vi "equilibrium_measurements_autofocus_build_brute_force.vi"() -> ()   [LabVIEW 2019]
uses:
  <vilib>/userDefined/High Color/IMAQdx.ctl
  <vilib>/vision/driver/IMAQdx.llb/IMAQdx Attribute Type.ctl
  <vilib>/vision/Management.llb/Cast Image 2 Method.ctl
  <vilib>/DAQmx/write.llb/DAQmx Write (Digital Bool 1Line 1Point).vi
  <vilib>/DAQmx/write.llb/DAQmx Write (Analog DBL 1Chan 1Samp).vi
  <vilib>/DAQmx/read.llb/DAQmx Read (Analog DBL 1Chan 1Samp).vi
  <vilib>/Analysis/baseanly.llb/Mean (DBL).vi
  <vilib>/DAQmx/create/channels.llb/DAQmx Create Channel (AO-Voltage-Basic).vi
  <vilib>/DAQmx/miscellaneous.llb/DAQmx Fill In Error Info.vi
  <vilib>/DAQmx/create/channels.llb/DAQmx Create Channel (AI-Temperature-Thermocouple).vi
  <vilib>/DAQmx/create/channels.llb/DAQmx Create Channel (CO-Pulse Generation-Frequency).vi
  <vilib>/DAQmx/configure/timing.llb/DAQmx Timing (Implicit).vi
  <vilib>/DAQmx/create/channels.llb/DAQmx Create Channel (DO-Digital Output).vi
  <vilib>/vision/driver/NI_Vision_Acquisition_Software.lvlib
  <resource>/objmgr/imaqdx.rc
  <vilib>/vision/NI_Vision_Development_Module.lvlib
  <vilib>/Analysis/NI_AALBase.lvlib
  <resource>/objmgr/daqmx.rc
panel:
  in  "Execute autofocus":bool=TRUE
  in  "Step Signal \nOutput Line 3":tag="/Dev3/PFI2"
  in  "Step Pulse Train \nFrequency (Hz) 3":dbl=200.0 format="%.6f"
  in  "Step Signal \nOutput Line 2":tag="/Dev3/PFI2"
  in  "Step Pulse Train \nFrequency (Hz) 2":dbl=200.0 format="%.6f"
  out "Direction":bool
  in  "Direction Line":tag="Dev3/port1/line4"
  in  "Enable Drive":bool
  in  "Enable Line":tag="Dev3/port1/line1"
  in  "Step Signal \nOutput Line":tag="/Dev3/PFI2"
  in  "Step Pulse Train \nFrequency (Hz)":dbl=200.0 format="%.6f"
  out "Video":bool
  in  "Action":i32(listbox)
  out "meanIntensity":dbl[](array[numeric])
  out "varLaplacian":dbl[](array[numeric])
  out "mean":dbl
  out "variance":dbl
  out "Avg Intensity":dbl(graph)=4.716017316017316
  in  "Monitor focus":bool
  out "?":dbl(graph)=701.3672509340029
  in  "ROI":T1={"Global Rectangle"=[], "Contours"=[{"Contour Type"=0, "ROI Type"=3, "Points"=[231, 86, 235, 90]}, {"Contour Type"=0, "ROI Type"=3, "Points"=[193, 50, 270, 125]}]}
  in  "error in":errorcluster
  in  "File path for video":string="C:\\Users\\Aniket\\Desktop\\mCherry_calibration\\new_lens\\laser_calibration\\laser_and_heating\\"
  in  "Laser profile file path":path=path "C:/Users/Aniket/Desktop/mCherry_calibration/new_lens/laser_calibration/laser_profiles/new_profile.txt"
  in  "Trigger Laser":bool
  in  "Power Generator":refnum<visa-resource-name>="COM3"
  in  "Desired \nTemperature":dbl=20.0 format="%#_13g"
  in  "PID Control":bool
  in  "Image file path \n(Do not add specify file extension - set to png)":path=path "C:/Users/Aniket/Desktop/mCherry_calibration/new_lens/laser_calibration/laser_profiles.txt"
  out "Current \nTemperature":dbl format="%0.2f"
  out "?":dbl[](graph)=[37.63236695538445]
  out "error out 7":errorcluster
  out "error out 6":errorcluster
  out "error out 5":errorcluster
  out "Exposure Time":dbl
  in  "ON/OFF":bool
  out "error out 3":errorcluster
  in  "LED":dbl(slide) scale=0.0..10.0
  in  "Refresh":bool
  out "Record":bool
  out "Processed Frames per Second":dbl
  out "Acquired Frame Rate":dbl
  out "error out":errorcluster
  out "Camera Display":T2(plugin-control) caption="Image Out"
  in  "Frame Rate":dbl=20.0
  out "Attribute Information Array":T4(array[cluster])
  in  "Session In":T5="cam0"
  # "Spot motion"
  # "Stage motion"
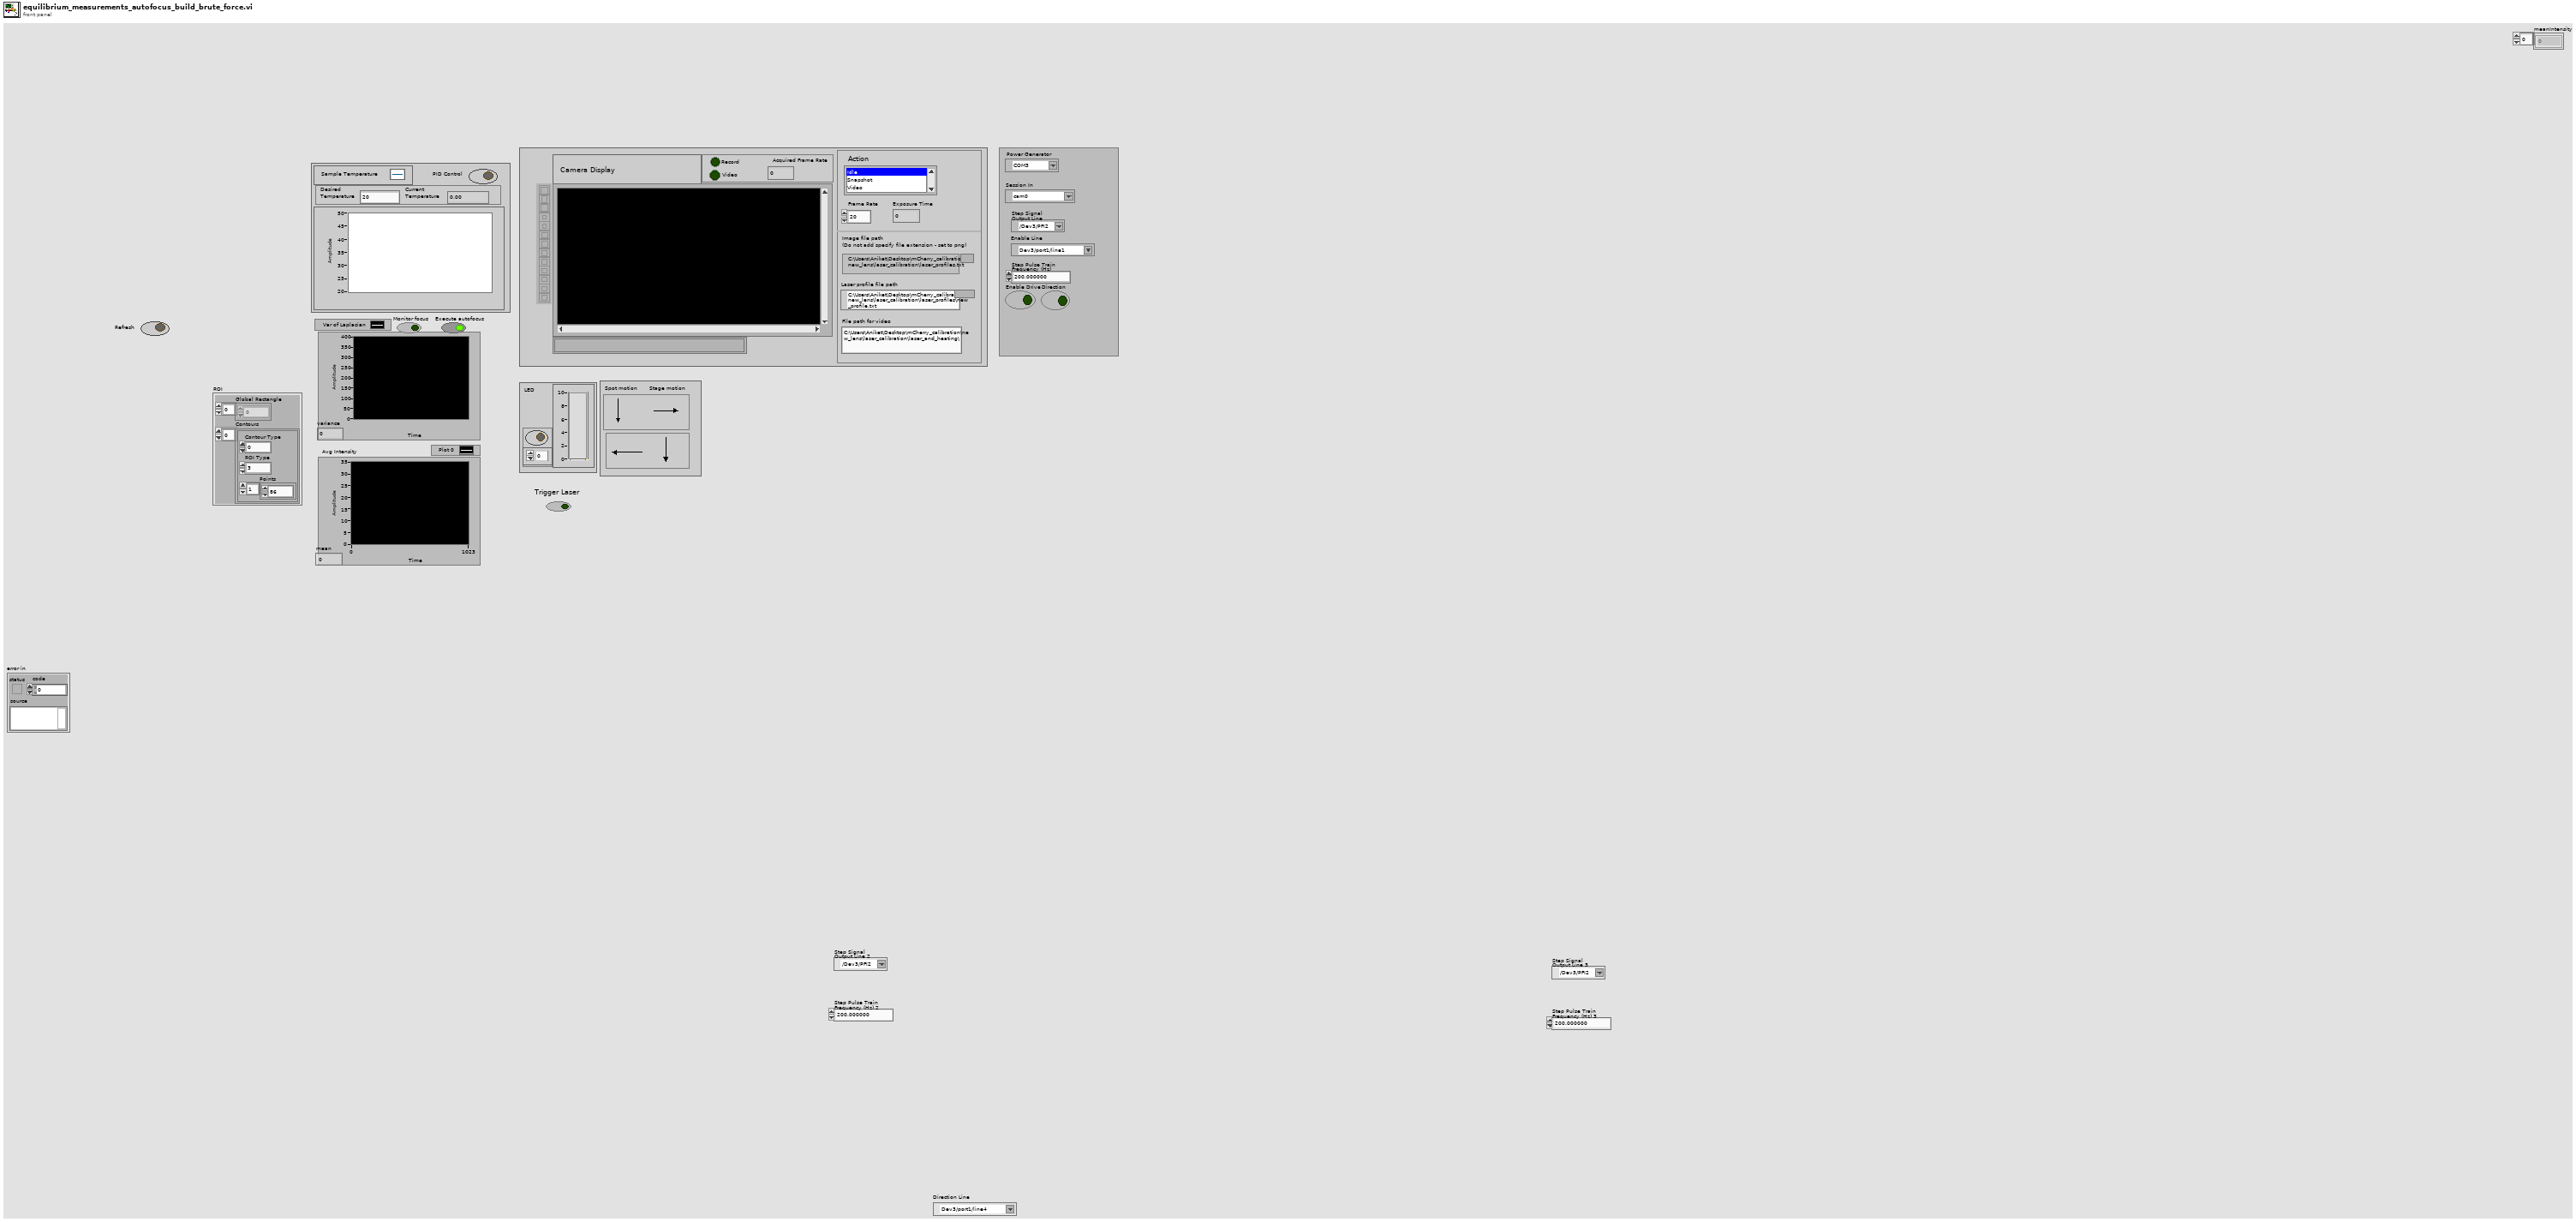
[diagram p1: front panel]
types:
  T1 = cluster{"Global Rectangle":i32[], "Contours":cluster{"Contour Type":u32, "ROI Type":u32, "Points":i32[]}[]}
  T2 = typedef "IMAQ Image.ctl" = refnum<image>
  T3 = typedef "NI_Vision_Acquisition_Software.lvlib/IMAQdx Attribute Type.ctl" = enum32{"U32", "I64", "DBL", "String", "Enum", "Bool", "Command"}
  T4 = cluster{"Attribute Type":T3, "Readable":bool, "Writable":bool, "Attribute Name":string}[]
  T5 = typedef "IMAQdx.ctl" = refnum<k21>
  T6 = typedef "Image Type" = u32
  T7 = typedef "ROI Descriptor" = cluster{"Global Rectangle":i32[], "Contours":cluster{"ID":enum32{"External", "Internal"}, "Type":u32, "Coordinates":i32[]}[]}
  T8 = typedef "IMAQ Rectangle" = cluster{"Left":i32, "Top":i32, "Right":i32, "Bottom":i32, "Rotation":dbl}
  T9 = cluster{"Mean Intensity":sgl, "Standard  Deviation":sgl, "Minimum Intensity":sgl, "Maximum Intensity":sgl}
  T10 = typedef "Cast Image 2 Method.ctl" = u32
  T11 = typedef "IMAQ AVI2 Refnum.ctl" = refnum<k20>
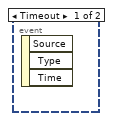
[diagram p3: hidden frame]
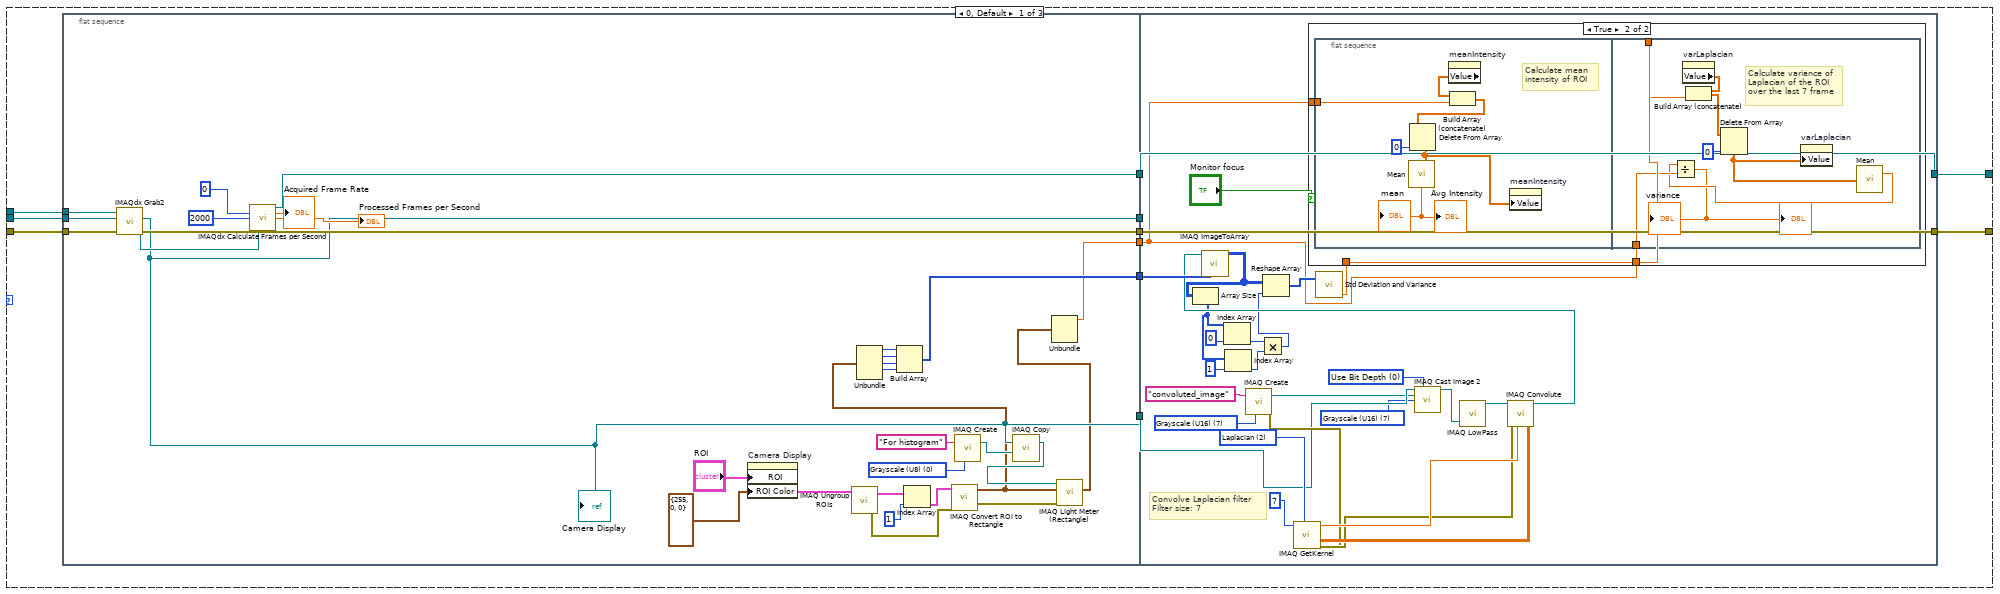
[diagram p6: hidden frame]
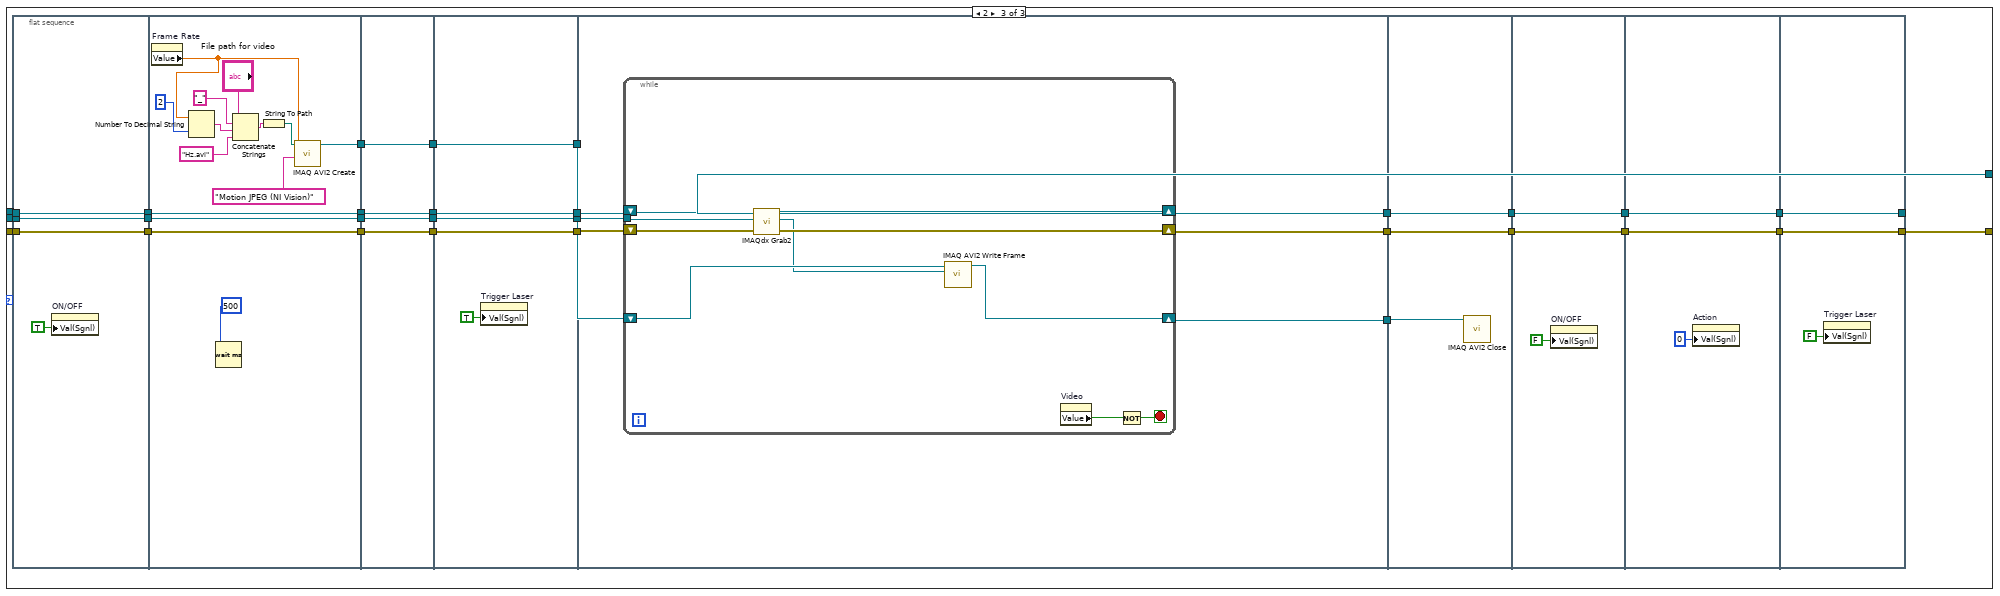
[diagram p8: hidden frame]
diagram:
  w12 = 10200 items=["Built-In"=10200, "Constant Value"=10116, "Channel"=10113]  # cjc source
  w14 = ""  # cjc channel
  w15 = 25.0  # cjc value
  w16 = 10072 items=["J"=10072, "K"=10073, "N"=10077, "R"=10082, "S"=10085, "T"=10086, "B"=10047, "E"=10055]  # thermocouple type
  w17 = 10143 items=["deg C"=10143, "deg F"=10144, "Kelvins"=10325, "deg R"=10145, "From Custom Scale"=10065]  # units
  w13 = "Temperature"  # channel name
  w18 = 0.0  # minimum value
  w19 = 100.0  # maximum value
  w21 = TRUE  # auto cleanup
  w44 = 10348 items=["Volts"=10348, "From Custom Scale"=10065] ("units")
  w46 = -1 items=["Default"=-1, "RSE"=10083, "NRSE"=10078, "Differential"=10106, "Pseudodifferential"=12529] ("input terminal configuration")
  w58 = T6 0 items=["Grayscale (U8)", "Grayscale (I16)", "Grayscale (SGL)", "Complex (CSG)", "RGB (U32)", "HSL (U32)", "RGB (U64)", "Grayscale (U16)"] ("Image Type")
  # "Total displacement of the objective from the origin\nMonitoring displacement allows keeping the search\nwithin a fixed range from the origin, to make sure\nthe objective does not drift too far"
  # "Set maximum exposure time \npermissible by the current frame rate"
  # "Excitation LED Control"
  # "Temperature measurement using thermocouple"
  # "PID Controller"
  # "Initialize arrays for focus detection"
  # "This array stores mean intensity in the last 10 frames\nInitiated as zeros"
  # "This array stores variance of Laplacian in the last 10 frames\nInitiated as zeros"
  n1 = call <vilib>:"DAQmx Create Task.vi"("auto cleanup"=w21, "error in"="error in") -> ("task out"=w20:refnum<k21>, "error out"=w22:errorcluster)  [unwired: 12 in]
  n2 = call-poly <vilib>:"DAQmx Create Virtual Channel.vi"("task in"=w20, "maximum value"=w19, "minimum value"=w18, "physical channels"=tag "Dev1/ai0", "cjc source"=w12, "name to assign"=w13, "units"=w17, "cjc channel"=w14, "error in"=w22, "thermocouple type"=w16, "cjc value"=w15) -> ("task out"=w11:refnum<k21>, "error out"=w10:errorcluster)  [unwired: 3 in]
  "error out 7" <- w10
  n3 = call-poly <vilib>:"DAQmx Create Virtual Channel.vi"("maximum value"=10.0, "minimum value"=0.0, "output terminal configuration"=w46, "physical channels"=tag "Dev3/ao0", "name to assign"="LED", "units"=w44) -> ("task out"=w42:refnum<k21>, "error out"=w41:errorcluster)  [unwired: 8 in]
  n4 = call <vilib>:"DAQmx Start Task.vi"("task/channels in"=w42, "error in"=w41) -> ("task out"=w40:refnum<k21>, "error out"=w39:errorcluster)  [unwired: 12 in]
  n5 = while {
    tunnel: w11 -> [w71]
    tunnel: w10 -> [w70]
    tunnel: [w69] -> w26
    tunnel: [w68] -> w25
    stop <- FALSE ("Monitor Temperature") stop-if-true
    n6 = Wait Until Next ms Multiple(millisecond multiple=u32 1000 ("millisecond timer value")) -> ()  [unwired: 1 out]
    n7 = call-poly <vilib>:"DAQmx Read.vi"("task/channels in"=w71, "error in"=w70) -> ("task out"=w69:refnum<k21>, "data"=w65:dbl, "error out"=w68:errorcluster)  [unwired: 11 in]
    n8 = Build Array(w65) -> (→"?":dbl[])
    n9 = Multiply(x=w65, y=1.07) -> (x*y=w63:dbl)
    n10 = Subtract(x=w63, y=2.74) -> (x-y=→"Current \nTemperature":dbl)
  }
  n11 = while {
    shift-right: [w75] -> w38
    shift-left: w40 -> [w77]
    shift-right: [w74] -> w37
    shift-left: w39 -> [w76]
    stop <- FALSE stop-if-true
    n12 = event shown="[0] \"LED\", \"ON/OFF\": Value Change" {
      selector: _ -> [_]
      dyn-events: _ -> [_]
      timeout: _ -> [_]
      tunnel: w77 -> [w86]
      tunnel: w76 -> [w85]
      tunnel: [w84] -> w75
      tunnel: [w83] -> w74
      event "LED", "ON/OFF": Value Change {
        n13 = event-data() -> ()  [unwired: 1 in, 6 out]
        n14 = Boolean To (0,1)(Boolean="ON/OFF") -> (0, 1=w79:i16)
        n15 = Multiply(x="LED", y=w79) -> (x*y=w78:dbl)
        n16 = call-poly <vilib>:"DAQmx Write.vi"("task/channels in"=w86, "auto start"=TRUE, "data"=w78, "error in"=w85) -> ("task out"=w84:refnum<k21>, "error out"=w83:errorcluster)  [unwired: 9 in, 1 out]
      }
    }
  }
  n17 = call "IMAQ Create"("Image Name"="Live", "Image Type"=w58) -> ("New Image"=w52:T2, "error out"=w51:errorcluster)  [unwired: 3 in]
  n18 = call <vilib>:"DAQmx Stop Task.vi"("task/channels in"=w26, "error in"=w25) -> ("error out"=→"error out 6":errorcluster)  [unwired: 12 in, 1 out]
  n19 = call <vilib>:"DAQmx Stop Task.vi"("task/channels in"=w38, "error in"=w37) -> ("error out"=→"error out 3":errorcluster)  [unwired: 12 in, 1 out]
  n20 = call <vilib>:"IMAQdx Open Camera.vi"("error in"=w51, "Session In"="Session In") -> ("error out"=w56:errorcluster, "Session Out"=w57:T5)  [unwired: 8 in]
  "error out 5" <- w56
  n21 = call <vilib>:"IMAQdx Enumerate Attributes.vi"("error in"=w56, "Session In"=w57) -> ("Attribute Information Array"=→"Attribute Information Array":T4)  [unwired: 7 in, 2 out]
  n22 = while {
    stop <- FALSE stop-if-true
    n23 = event shown="[1] \"Trigger Laser\": Value Change" {
      selector: _ -> [_ _]
      dyn-events: _ -> [_ _]
      timeout: _ -> [_ _]
      event Timeout {
        n24 = event-data() -> ()  [unwired: 1 in, 3 out]
      }
      event "Trigger Laser": Value Change {
        n25 = event-data() -> ()  [unwired: 1 in, 6 out]
        n26 = property on="Action" class="LstBox (strict)"() -> ("Value"=w88:i32)  [unwired: 2 in, 2 out]
        n27 = case shown="2" w88 {
          frame 0, Default {
          }
          frame 1 {
          }
          frame 2 {
            n28 = flat-sequence {
              frame #0 {
                "Video" <- TRUE ("Video")
              }
              frame #1 {
                # "Read voltage values for\nlaser control from a text file"
                n29 = Read from Text File(file (use dialog)="Laser profile file path") -> (text=w97:string)  [unwired: 3 in, 3 out]
                n30 = Spreadsheet String To Array(delimiter (Tab)="\r\n", format string="%f", spreadsheet string=w97, array type (2D Dbl)=dbl[][] []) -> (array=w99:dbl[][])
                n31 = Array Size(array=w99) -> (size(s)=w98:i32[])
                n32 = Index Array(array=w98, index=0) -> (element=w101:i32)
                n33 = Reshape Array(w99, w101) -> (w100:dbl[])
                n34 = call "Untitled 43.vi"() -> ("error out"=w90:errorcluster, "task out"=w91:refnum<k21>)  [unwired: 10 in]
                n35 = for {
                  N: w101 -> [_]
                  tunnel: w100 -> [w102] mode=indexing
                  tunnel: w91 -> [w104]
                  tunnel: w90 -> [w103]
                  w105 = TRUE  # auto start
                  n36 = Wait (ms)(milliseconds to wait=u32 10) -> ()  [unwired: 1 out]
                  n37 = call-poly <vilib>:"DAQmx Write.vi"("task/channels in"=w104, "auto start"=w105, "data"=w102, "error in"=w103) -> ()  [unwired: 9 in, 3 out]
                }
              }
              frame #2 {
                n38 = property on="Video" class="Bool (strict)"("Val(Sgnl)"=FALSE ("Value (Signaling)")) -> ()  [unwired: 2 in, 2 out]
              }
            }
          }
        }
      }
    }
  }
  n39 = while {
    stop <- FALSE stop-if-true
    n40 = local read "Current \nTemperature"() -> (w111:dbl)
    n41 = call "IronFishPIDtakeCurrentTemp.vi"(0:"Power Generator", "Switch"="PID Control", "Desired Temp"="Desired \nTemperature", "Current Temp"=w111) -> ()  [unwired: 4 in, 1 out]
  }
  n42 = while {
    stop <- FALSE stop-if-true
    n43 = event shown="[0] \"Execute autofocus\": Value Change" {
      selector: _ -> [_]
      dyn-events: _ -> [_]
      timeout: _ -> [_]
      event "Execute autofocus": Value Change {
        n44 = event-data() -> ()  [unwired: 1 in, 6 out]
        n45 = property on="Execute autofocus" class="Bool (strict)"() -> ("Value"=w114:bool)  [unwired: 2 in, 2 out]
        n46 = case shown="True" w114 {
          frame False {
          }
          frame True {
            # "Generate continuous samples for constant velocity, or finite \nsamples to move the motor a finite number of steps."
            # "Default is the\nobjective going\ndownwards"
            n47 = flat-sequence {
              tunnel: [w191] -> w117
              tunnel: w117 -> [w224]
              tunnel: [w224] -> w116
              tunnel: w116 -> [w226]
              frame #0 {
                n48 = flat-sequence {
                  tunnel: [w163] -> w158
                  tunnel: [w162] -> w157
                  tunnel: [w161] -> w154
                  tunnel: w158 -> [w183]
                  tunnel: w157 -> [w182]
                  tunnel: [w181] -> w156
                  tunnel: [w180] -> w155
                  tunnel: w154 -> [w179]
                  tunnel: w156 -> [w185]
                  tunnel: w155 -> [w184]
                  frame #0 {
                    n49 = property on="Direction" class="Bool (strict)"("Value"=FALSE ("Direction")) -> ()  [unwired: 2 in, 2 out]
                    n50 = Wait (ms)(milliseconds to wait=u32 50) -> ()  [unwired: 1 out]
                  }
                  frame #1 {
                    w164 = 150 ("samples per channel")
                    w176 = 10178 items=["Finite Samples"=10178, "Continuous Samples"=10123, "Hardware Timed Single Point"=12522] ("sample mode")
                    n51 = call-poly <vilib>:"DAQmx Create Virtual Channel.vi"("frequency"="Step Pulse Train \nFrequency (Hz) 2", "counter"=tag "Dev3/ctr0") -> ("task out"=w172:refnum<k21>, "error out"=w171:errorcluster)  [unwired: 12 in]
                    n52 = property class="DAQmx Channel"(reference=w172, error in=w171, "CO.Pulse.Term"="Step Signal \nOutput Line 2") -> (reference out=w175:refnum<k21>, error out=w174:errorcluster)
                    n53 = Divide(x=1000.0, y="Step Pulse Train \nFrequency (Hz) 2") -> (x/y=w167:dbl)
                    n54 = Multiply(x=w167, y=w164) -> (x*y=w169:dbl)
                    n55 = Add(x=w169, y=5.0) -> (x+y=w161:dbl)
                    n56 = call-poly <vilib>:"DAQmx Timing.vi"("task/channels in"=w175, "sample mode"=w176, "samples per channel"=w164, "error in"=w174) -> ("task out"=w178:refnum<k21>, "error out"=w177:errorcluster)  [unwired: 10 in]
                    n57 = call <vilib>:"DAQmx Start Task.vi"("task/channels in"=w178, "error in"=w177) -> ("task out"=w163:refnum<k21>, "error out"=w162:errorcluster)  [unwired: 12 in]
                  }
                  frame #2 {
                    n58 = call <vilib>:"DAQmx Is Task Done.vi"("task/channels in"=w183, "error in"=w182) -> ("task out"=w180:refnum<k21>, "error out"=w181:errorcluster)  [unwired: 11 in, 1 out]
                    n59 = Wait (ms)(milliseconds to wait=w179) -> ()  [unwired: 1 out]
                  }
                  frame #3 {
                    n60 = call <vilib>:"DAQmx Stop Task.vi"("task/channels in"=w184, "error in"=w185) -> ("task out"=w188:refnum<k21>, "error out"=w186:errorcluster)  [unwired: 12 in]
                    n61 = call <vilib>:"DAQmx Clear Task.vi"("task in"=w188, "error in"=w186) -> ("error out"=w187:errorcluster)  [unwired: 13 in]
                    n62 = call <vilib>:"Simple Error Handler.vi"("error in (no error)"=w187) -> ()  [unwired: 4 in, 5 out]
                  }
                }
              }
              frame #1 {
                n63 = property on="Direction" class="Bool (strict)"("Value"=TRUE ("Direction")) -> ()  [unwired: 2 in, 2 out]
                n64 = Wait (ms)(milliseconds to wait=u32 50) -> ()  [unwired: 1 out]
              }
              frame #2 {
                # "Note that coincidentally,\nthe gradient and the number\nof steps is numerically the same"
                n65 = for {
                  N: 450 -> [_]
                  tunnel: [w196] -> w194 mode=indexing
                  n66 = flat-sequence {
                    tunnel: [w221] -> w196
                    frame #0 {
                      w211 = 10178 items=["Finite Samples"=10178, "Continuous Samples"=10123, "Hardware Timed Single Point"=12522] ("sample mode")
                      n67 = call-poly <vilib>:"DAQmx Create Virtual Channel.vi"("frequency"="Step Pulse Train \nFrequency (Hz)", "counter"=tag "Dev3/ctr0") -> ("task out"=w203:refnum<k21>, "error out"=w202:errorcluster)  [unwired: 12 in]
                      n68 = Divide(x=1000.0, y="Step Pulse Train \nFrequency (Hz)") -> (x/y=w206:dbl)
                      n69 = property class="DAQmx Channel"(reference=w203, error in=w202, "CO.Pulse.Term"="Step Signal \nOutput Line") -> (reference out=w210:refnum<k21>, error out=w209:errorcluster)
                      n70 = Multiply(x=w206, y=1.0) -> (x*y=w208:dbl)
                      n71 = Add(x=w208, y=2.0) -> (x+y=w214:dbl)
                      n72 = Wait (ms)(milliseconds to wait=w214) -> ()  [unwired: 1 out]
                      n73 = call-poly <vilib>:"DAQmx Timing.vi"("task/channels in"=w210, "sample mode"=w211, "samples per channel"=1, "error in"=w209) -> ("task out"=w213:refnum<k21>, "error out"=w212:errorcluster)  [unwired: 10 in]
                      n74 = call <vilib>:"DAQmx Start Task.vi"("task/channels in"=w213, "error in"=w212) -> ("task out"=w216:refnum<k21>, "error out"=w215:errorcluster)  [unwired: 12 in]
                      n75 = call <vilib>:"DAQmx Is Task Done.vi"("task/channels in"=w216, "error in"=w215) -> ("task out"=w219:refnum<k21>, "error out"=w218:errorcluster)  [unwired: 11 in, 1 out]
                      n76 = call <vilib>:"DAQmx Stop Task.vi"("task/channels in"=w219, "error in"=w218) -> ("task out"=w220:refnum<k21>, "error out"=w217:errorcluster)  [unwired: 12 in]
                      n77 = call <vilib>:"DAQmx Clear Task.vi"("task in"=w220, "error in"=w217) -> ("error out"=w198:errorcluster)  [unwired: 13 in]
                      n78 = call <vilib>:"Simple Error Handler.vi"("error in (no error)"=w198) -> ()  [unwired: 4 in, 5 out]
                    }
                    frame #1 {
                      n79 = property on="variance" class="DigNum (strict)"() -> ("Value"=w221:dbl)  [unwired: 2 in, 2 out]
                    }
                  }
                }
                n80 = Array Max & Min(array=w194) -> (max index (indices)=w193:i32)  [unwired: 3 out]
                n81 = Subtract(x=449, y=w193) -> (x-y=w191:i32)
              }
              frame #3 {
                n82 = property on="Direction" class="Bool (strict)"("Value"=FALSE ("Direction")) -> ()  [unwired: 2 in, 2 out]
                n83 = Wait (ms)(milliseconds to wait=u32 50) -> ()  [unwired: 1 out]
              }
              frame #4 {
                # "offset"
                n84 = flat-sequence {
                  tunnel: w227 -> [w236]
                  tunnel: [w235] -> w232
                  tunnel: [w234] -> w231
                  tunnel: [w233] -> w228
                  tunnel: w232 -> [w255]
                  tunnel: w231 -> [w254]
                  tunnel: [w253] -> w230
                  tunnel: [w252] -> w229
                  tunnel: w228 -> [w251]
                  tunnel: w230 -> [w257]
                  tunnel: w229 -> [w256]
                  frame #0 {
                    w248 = 10178 items=["Finite Samples"=10178, "Continuous Samples"=10123, "Hardware Timed Single Point"=12522] ("sample mode")
                    n85 = call-poly <vilib>:"DAQmx Create Virtual Channel.vi"("frequency"="Step Pulse Train \nFrequency (Hz) 3", "counter"=tag "Dev3/ctr0") -> ("task out"=w240:refnum<k21>, "error out"=w239:errorcluster)  [unwired: 12 in]
                    n86 = Divide(x=1000.0, y="Step Pulse Train \nFrequency (Hz) 3") -> (x/y=w243:dbl)
                    n87 = property class="DAQmx Channel"(reference=w240, error in=w239, "CO.Pulse.Term"="Step Signal \nOutput Line 3") -> (reference out=w247:refnum<k21>, error out=w246:errorcluster)
                    n88 = Multiply(x=w243, y=w236) -> (x*y=w245:dbl)
                    n89 = Add(x=w245, y=5.0) -> (x+y=w233:dbl)
                    n90 = call-poly <vilib>:"DAQmx Timing.vi"("task/channels in"=w247, "sample mode"=w248, "samples per channel"=w236, "error in"=w246) -> ("task out"=w250:refnum<k21>, "error out"=w249:errorcluster)  [unwired: 10 in]
                    n91 = call <vilib>:"DAQmx Start Task.vi"("task/channels in"=w250, "error in"=w249) -> ("task out"=w235:refnum<k21>, "error out"=w234:errorcluster)  [unwired: 12 in]
                  }
                  frame #1 {
                    n92 = call <vilib>:"DAQmx Is Task Done.vi"("task/channels in"=w255, "error in"=w254) -> ("task out"=w253:refnum<k21>, "error out"=w252:errorcluster)  [unwired: 11 in, 1 out]
                    n93 = Wait (ms)(milliseconds to wait=w251) -> ()  [unwired: 1 out]
                  }
                  frame #2 {
                    n94 = call <vilib>:"DAQmx Stop Task.vi"("task/channels in"=w257, "error in"=w256) -> ("task out"=w260:refnum<k21>, "error out"=w259:errorcluster)  [unwired: 12 in]
                    n95 = call <vilib>:"DAQmx Clear Task.vi"("task in"=w260, "error in"=w259) -> ("error out"=w258:errorcluster)  [unwired: 13 in]
                    n96 = call <vilib>:"Simple Error Handler.vi"("error in (no error)"=w258) -> ()  [unwired: 4 in, 5 out]
                  }
                }
                n97 = Subtract(x=w226, y=20) -> (x-y=w227:i32)
              }
              frame #5 {
                n98 = property on="Execute autofocus" class="Bool (strict)"("Val(Sgnl)"=FALSE ("Value (Signaling)")) -> ()  [unwired: 2 in, 2 out]
              }
            }
            n99 = while {
              stop <- w118 stop-if-true
              (unwired) FALSE
              w121 = 0 items=["one channel for each line", "one channel for all lines"] ("line grouping")
              w120 = 0 items=["one channel for each line", "one channel for all lines"] ("line grouping")
              # "Direction Line"
              # "Enable lines"
              n100 = call-poly <vilib>:"DAQmx Create Virtual Channel.vi"("lines"="Enable Line", "line grouping"=w120) -> ("task out"=w134:refnum<k21>, "error out"=w135:errorcluster)  [unwired: 12 in]
              n101 = call-poly <vilib>:"DAQmx Create Virtual Channel.vi"("lines"="Direction Line", "line grouping"=w121) -> ("task out"=w130:refnum<k21>, "error out"=w131:errorcluster)  [unwired: 12 in]
              n102 = flat-sequence {
                tunnel: w130 -> [w144]
                tunnel: w131 -> [w143]
                tunnel: [w142] -> w139
                tunnel: [w141] -> w138
                tunnel: [w152] -> w133
                tunnel: [w153] -> w132
                tunnel: w139 -> [w153]
                tunnel: w138 -> [w152]
                tunnel: w134 -> [w149]
                tunnel: w135 -> [w148]
                tunnel: [w147] -> w136
                tunnel: [w146] -> w137
                frame #0 {
                  n103 = property on="Direction" class="Bool (strict)"() -> ("Value"=w140:bool)  [unwired: 2 in, 2 out]
                  n104 = call-poly <vilib>:"DAQmx Write.vi"("task/channels in"=w144, "auto start"=TRUE, "data"=w140, "error in"=w143) -> ("task out"=w142:refnum<k21>, "error out"=w141:errorcluster)  [unwired: 9 in, 1 out]
                }
                frame #1 {
                  n105 = call-poly <vilib>:"DAQmx Write.vi"("task/channels in"=w149, "auto start"=TRUE, "data"="Enable Drive", "error in"=w148) -> ("task out"=w147:refnum<k21>, "error out"=w146:errorcluster)  [unwired: 9 in, 1 out]
                }
              }
              n106 = call <vilib>:"DAQmx Stop Task.vi"("task/channels in"=w136, "error in"=w137) -> ("task out"=w123:refnum<k21>, "error out"=w124:errorcluster)  [unwired: 12 in]
              n107 = property on="Execute autofocus" class="Bool (strict)"() -> ("Value"=w119:bool)  [unwired: 2 in, 2 out]
              n108 = call <vilib>:"DAQmx Stop Task.vi"("task/channels in"=w132, "error in"=w133) -> ("task out"=w129:refnum<k21>, "error out"=w128:errorcluster)  [unwired: 12 in]
              n109 = call <vilib>:"DAQmx Clear Task.vi"("task in"=w123, "error in"=w124) -> ("error out"=w125:errorcluster)  [unwired: 13 in]
              n110 = Not(x=w119) -> (.not. x?=w118:bool)
              n111 = call <vilib>:"DAQmx Clear Task.vi"("task in"=w129, "error in"=w128) -> ("error out"=w127:errorcluster)  [unwired: 13 in]
              n112 = call <vilib>:"Simple Error Handler.vi"("error in (no error)"=w127) -> ()  [unwired: 4 in, 5 out]
              n113 = call <vilib>:"Simple Error Handler.vi"("error in (no error)"=w125) -> ()  [unwired: 4 in, 5 out]
            }
            "Direction" <- FALSE ("Clockwise/Counterclockwise?")
          }
        }
      }
    }
  }
  n114 = call <vilib>:"IMAQdx Configure Grab.vi"("error in"=w56, "Session In"=w57) -> ("error out"=w54:errorcluster, "Session Out"=w35:T5)  [unwired: 8 in]
  n115 = while {
    stop <- FALSE stop-if-true
    n116 = event shown="[0] \"Refresh\": Value Change" {
      selector: _ -> [_]
      dyn-events: _ -> [_]
      timeout: _ -> [_]
      event "Refresh": Value Change {
        (unwired) dbl[] [] ("History Data")
        n117 = event-data() -> ()  [unwired: 1 in, 4 out]
      }
    }
  }
  n118 = property class="IMAQdx"(reference=w35, error in=w54, "ActiveAttribute"="CameraAttributes::AcquisitionControl::AcquisitionFrameRate", "ValueDBL"="Frame Rate") -> (reference out=w30:T5, error out=w28:errorcluster)
  n119 = local write "Frame Rate"("Frame Rate") -> ()
  n120 = local read "Frame Rate"() -> (w32:dbl)
  n121 = Divide(x=991000.0, y=w32) -> (x/y=w31:dbl)
  "Exposure Time" <- w31
  n122 = property class="IMAQdx"(reference=w30, error in=w28, "ActiveAttribute"="CameraAttributes::AcquisitionControl::ExposureTime", "ValueDBL"=w31) -> (reference out=w29:T5, error out=w27:errorcluster)
  n123 = property on="Action" class="LstBox (strict)"("Val(Sgnl)"=0 ("Value (Signaling)")) -> ()  [unwired: 2 in, 2 out]
  n124 = while {
    tunnel: w29 -> [w269]
    tunnel: w52 -> [w267]
    shift-right: [w266] -> w50
    shift-left: w27 -> [w268]
    tunnel: [w263] -> w2
    stop <- FALSE ("Stop") stop-if-true
    n125 = case shown="1" "Action" {
      tunnel: w269 -> [w280 w372 w443]
      tunnel: w268 -> [w279 w374 w441]
      tunnel: w267 -> [w278 w373 w442]
      tunnel: [w277 w375 w439] -> w266
      tunnel: [w276 w376 w440] -> w263
      frame 0, Default {
        n126 = flat-sequence {
          tunnel: w280 -> [w310]
          tunnel: w279 -> [w309]
          tunnel: w278 -> [w308]
          tunnel: [w307] -> w275
          tunnel: [w305] -> w274
          tunnel: [w292] -> w273
          tunnel: [w292] -> w272
          tunnel: [w284] -> w271
          tunnel: [w281] -> w270
          tunnel: [w338] -> w276
          tunnel: [w339] -> w277
          tunnel: w275 -> [w339]
          tunnel: w274 -> [w338]
          tunnel: w273 -> [_]
          tunnel: w272 -> [w320]
          tunnel: w271 -> [w329]
          tunnel: w270 -> [w311]
          frame #0 {
            w293 = T6 0 items=["Grayscale (U8)", "Grayscale (I16)", "Grayscale (SGL)", "Complex (CSG)", "RGB (U32)", "HSL (U32)", "RGB (U64)", "Grayscale (U16)"] ("Image Type")
            n127 = call <vilib>:"IMAQdx Grab2.vi"("error in"=w309, "Image In"=w308, "Session In"=w310) -> ("error out"=w307:errorcluster, "Image Out"=w292:T2, "Session Out"=w306:T5)  [unwired: 5 in, 1 out]
            "Camera Display" <- w292
            n128 = call <vilib>:"IMAQdx Calculate Frames per Second.vi"("Session In"=w306, "Buffer Number"=u32 0, "Minimum Display Update Interval (ms)"=u32 2000) -> ("Session Out"=w305:T5, "Acquired Frames per Second"=→"Acquired Frame Rate":dbl, "Processed Frames per Second"=→"Processed Frames per Second":dbl)  [unwired: 6 in, 4 out]
            n129 = property on="Camera Display" class="ImageControl"("ROI"="ROI", "ROI Color"=cluster{"Red":u8, "Green":u8, "Blue":u8} {"Red"=255, "Green"=0, "Blue"=0}) -> ()  [unwired: 2 in, 2 out]
            n130 = call "IMAQ Ungroup ROIs"("ROI Descriptor"="ROI") -> ("error out"=w296:errorcluster, "ROI Descriptors out"=w299:T7[])  [unwired: 3 in]
            n131 = Index Array(array=w299, index=1) -> (element=w297:T7)
            n132 = call "IMAQ Convert ROI to Rectangle"("error in (no error)"=w296, "ROI Descriptor"=w297) -> ("error out"=w295:errorcluster, "Rectangle"=w289:T8)  [unwired: 7 in]
            n133 = Unbundle(w289) -> ("Left"=w288:i32, "Top"=w287:i32, "Right"=w286:i32, "Bottom"=w285:i32)  [unwired: 1 out]
            n134 = Build Array(w288, w287, w286, w285) -> (w284:i32[])
            n135 = call "IMAQ Create"("Image Name"="For histogram", "Image Type"=w293) -> ("New Image"=w291:T2)  [unwired: 3 in, 1 out]
            n136 = call "IMAQ Copy"("Image Dst"=w291, "Image Src"=w292) -> ("Image Dst Out"=w290:T2)  [unwired: 4 in, 1 out]
            n137 = call "IMAQ Light Meter (Rectangle)"("error in (no error)"=w295, "Rectangle"=w289, "Image"=w290) -> ("Gray Level Intensities"=w282:T9)  [unwired: 4 in, 4 out]
            n138 = Unbundle(w282) -> ("Mean Intensity"=w281:sgl)  [unwired: 3 out]
          }
          frame #1 {
            w316 = T6 7 items=["Grayscale (U8)", "Grayscale (I16)", "Grayscale (SGL)", "Complex (CSG)", "RGB (U32)", "HSL (U32)", "RGB (U64)", "Grayscale (U16)"] ("Image Type")
            w319 = T10 0 items=["Use Bit Depth", "Shift", "Use Lookup Table"] ("Method")
            w334 = u16 2 items=["Gradient"=1, "Laplacian"=2, "Smoothing"=3, "Gaussian"=4] ("Kernel Family")
            w336 = T6 7 items=["Grayscale (U8)", "Grayscale (I16)", "Grayscale (SGL)", "Complex (CSG)", "RGB (U32)", "HSL (U32)", "RGB (U64)", "Grayscale (U16)"] ("Image Type")
            # "Convolve Laplacian filter \nFilter size: 7"
            n139 = call "IMAQ Create"("Image Name"="convoluted_image", "Image Type"=w336) -> ("New Image"=w318:T2, "error out"=w330:errorcluster)  [unwired: 3 in]
            n140 = call "IMAQ GetKernel"("Kernel Family"=w334, "error in (no error)"=w330, "Kernel Size (3,5,...)"=7) -> ("error out"=w331:errorcluster, "Kernel"=w332:sgl[][], "Divider"=w333:sgl)  [unwired: 5 in, 1 out]
            n141 = call "IMAQ Cast Image 2"("Image Src"=w320, "Method"=w319, "Image Dst"=w318, "Image Type"=w316) -> ("Image Dst Out"=w317:T2)  [unwired: 10 in, 1 out]
            n142 = call "IMAQ LowPass"("Image Src"=w317) -> ("Image Dst Out"=w321:T2)  [unwired: 6 in, 1 out]
            n143 = call "IMAQ Convolute"("Kernel"=w332, "Divider (kernel sum)"=w333, "error in (no error)"=w331, "Image Src"=w321) -> ("Image Dst Out"=w328:T2)  [unwired: 6 in, 1 out]
            n144 = call "IMAQ ImageToArray"("Optional Rectangle"=w329, "Image"=w328) -> ("Image Pixels (U16)"=w312:u16[][])  [unwired: 2 in, 4 out]
            n145 = Array Size(array=w312) -> (size(s)=w315:i32[])
            n146 = Index Array(array=w315, index=0 ("index (row)")) -> (element=w325:i32)
            n147 = Index Array(array=w315, index=1) -> (element=w324:i32)
            n148 = Multiply(x=w325, y=w324) -> (x*y=w314:i32)
            n149 = Reshape Array(w312, w314) -> (w313:u16[])
            n150 = call <vilib>:"Std Deviation and Variance.vi"("X"=w313) -> ("variance"=w322:dbl)  [unwired: 1 in, 2 out]
            n151 = case shown="True" "Monitor focus" {
              tunnel: w322 -> [_ w342]
              tunnel: w311 -> [_ w341]
              tunnel: w311 -> [_ w340]
              frame False {
              }
              frame True {
                n152 = flat-sequence {
                  tunnel: w340 -> [w343]
                  tunnel: w342 -> [w352]
                  tunnel: w341 -> [w356]
                  frame #0 {
                    # "Calculate mean \nintensity of ROI"
                    n153 = property on="meanIntensity" class="Arr (strict)"() -> ("Value"=w346:dbl[])  [unwired: 2 in, 2 out]
                    n154 = Build Array (concatenate)(w346, w343) -> (w345:dbl[])
                    n155 = Delete From Array(array=w345, index=0) -> (array with subset deleted=w344:dbl[])  [unwired: 1 in, 1 out]
                    n156 = call-poly <vilib>:"Mean.vi"("X"=w344) -> ("mean"=→"Avg Intensity" →"mean":dbl)  [unwired: 1 out]
                    n157 = property on="meanIntensity" class="Arr (strict)"("Value"=w344) -> ()  [unwired: 2 in, 2 out]
                  }
                  frame #1 {
                    # "Calculate variance of\nLaplacian of the ROI\nover the last 7 frame"
                    n158 = property on="varLaplacian" class="Arr (strict)"() -> ("Value"=w353:dbl[])  [unwired: 2 in, 2 out]
                    n159 = Build Array (concatenate)(w353, w352) -> (w351:dbl[])
                    n160 = Delete From Array(array=w351, index=0) -> (array with subset deleted=w350:dbl[])  [unwired: 1 in, 1 out]
                    n161 = property on="varLaplacian" class="Arr (strict)"("Value"=w350) -> ()  [unwired: 2 in, 2 out]
                    n162 = call-poly <vilib>:"Mean.vi"("X"=w350) -> ("mean"=w355:dbl)  [unwired: 1 out]
                    n163 = Divide(x=w355, y=w356) -> (x/y=→"?" →"variance":dbl)
                  }
                }
              }
            }
          }
        }
      }
      frame 1 {
        n164 = flat-sequence {
          tunnel: w372 -> [w378]
          tunnel: w373 -> [w379]
          tunnel: w374 -> [w380]
          tunnel: [w380] -> w361
          tunnel: [w379] -> w360
          tunnel: [w378] -> w359
          tunnel: [w384] -> w367
          tunnel: [w383] -> w365
          tunnel: [w382] -> w363
          tunnel: w361 -> [w384]
          tunnel: w360 -> [w383]
          tunnel: w359 -> [w382]
          tunnel: w367 -> [w388]
          tunnel: [w388] -> w366
          tunnel: w365 -> [w387]
          tunnel: [w387] -> w364
          tunnel: w363 -> [w386]
          tunnel: [w386] -> w362
          tunnel: [w401] -> w371
          tunnel: [w405] -> w369
          tunnel: w366 -> [w404]
          tunnel: w364 -> [w403]
          tunnel: w362 -> [w402]
          tunnel: w371 -> [w408]
          tunnel: [w408] -> w370
          tunnel: w369 -> [w407]
          tunnel: [w407] -> w368
          tunnel: w370 -> [w411]
          tunnel: w368 -> [w410]
          tunnel: [w411] -> w358
          tunnel: [w410] -> w357
          tunnel: [w413] -> w375
          tunnel: [w414] -> w376
          tunnel: w358 -> [w414]
          tunnel: w357 -> [w413]
          frame #0 {
            "Record" <- TRUE ("Record")
          }
          frame #1 {
            n165 = property on="ON/OFF" class="Bool (strict)"("Val(Sgnl)"=TRUE ("ON/OFF")) -> ()  [unwired: 2 in, 2 out]
          }
          frame #2 {
            n166 = Wait (ms)(milliseconds to wait=u32 500) -> ()  [unwired: 1 out]
          }
          frame #3 {
            n167 = property on="Current \nTemperature" class="DigNum (strict)"() -> ("Value"=w399:dbl)  [unwired: 2 in, 2 out]
            n168 = Path To String(path="Image file path \n(Do not add specify file extension - set to png)") -> (string=w394:string)
            n169 = Number To Fractional String(number=w399, precision (6)=i16 2 ("width (-)")) -> (F-format string=w396:string)  [unwired: 2 in]
            n170 = Concatenate Strings("_" ("string"), w396) -> (w393:string)
            n171 = Concatenate Strings(w394, w393) -> (w392:string)
            n172 = call <vilib>:"IMAQdx Grab2.vi"("error in"=w404, "Image In"=w403, "Session In"=w402) -> ("error out"=w405:errorcluster, "Image Out"=w400:T2, "Session Out"=w401:T5)  [unwired: 5 in, 1 out]
            n173 = Concatenate Strings(w392, ".png" ("string")) -> (w390:string)
            n174 = String To Path(string=w390) -> (path=w389:path)
            n175 = call-poly "IMAQ Write File 2"("File Path"=w389, "Image"=w400) -> ()  [unwired: 8 in, 2 out]
          }
          frame #4 {
            n176 = property on="ON/OFF" class="Bool (strict)"("Val(Sgnl)"=FALSE ("ON/OFF")) -> ()  [unwired: 2 in, 2 out]
          }
          frame #5 {
            n177 = local write "Record"(FALSE ("Record")) -> ()
          }
          frame #6 {
            n178 = property on="Action" class="LstBox (strict)"("Val(Sgnl)"=0 ("Value (Signaling)")) -> ()  [unwired: 2 in, 2 out]
          }
        }
      }
      frame 2 {
        n179 = flat-sequence {
          tunnel: w441 -> [w445]
          tunnel: w442 -> [w446]
          tunnel: w443 -> [w447]
          tunnel: [w447] -> w438
          tunnel: [w446] -> w437
          tunnel: [w445] -> w436
          tunnel: w438 -> [w461]
          tunnel: [w461] -> w435
          tunnel: w437 -> [w460]
          tunnel: [w460] -> w433
          tunnel: w436 -> [w459]
          tunnel: [w459] -> w431
          tunnel: [w456] -> w424
          tunnel: w435 -> [w465]
          tunnel: [w465] -> w434
          tunnel: w433 -> [w464]
          tunnel: [w464] -> w432
          tunnel: w431 -> [w463]
          tunnel: [w463] -> w430
          tunnel: [w462] -> w425
          tunnel: w424 -> [w462]
          tunnel: w434 -> [w467]
          tunnel: w432 -> [w468]
          tunnel: w430 -> [w469]
          tunnel: [w469] -> w429
          tunnel: [w468] -> w428
          tunnel: [w467] -> w427
          tunnel: [w466] -> w426
          tunnel: w425 -> [w466]
          tunnel: w429 -> [w476]
          tunnel: w428 -> [w475]
          tunnel: w427 -> [w474]
          tunnel: [w472] -> w423
          tunnel: [w473] -> w422
          tunnel: [w477] -> w421
          tunnel: w426 -> [w471]
          tunnel: w423 -> [w490]
          tunnel: [w490] -> w418
          tunnel: w422 -> [w489]
          tunnel: [w489] -> w420
          tunnel: w421 -> [w488]
          tunnel: w420 -> [w493]
          tunnel: [w493] -> w419
          tunnel: w418 -> [w492]
          tunnel: [w492] -> w417
          tunnel: w419 -> [w495]
          tunnel: w417 -> [w496]
          tunnel: [w496] -> w416
          tunnel: [w495] -> w415
          tunnel: [w498] -> w439
          tunnel: [w499] -> w440
          tunnel: w416 -> [w499]
          tunnel: w415 -> [w498]
          frame #0 {
            n180 = property on="ON/OFF" class="Bool (strict)"("Val(Sgnl)"=TRUE ("Value (Signaling)")) -> ()  [unwired: 2 in, 2 out]
          }
          frame #1 {
            n181 = property on="Frame Rate" class="DigNum (strict)"() -> ("Value"=w454:dbl)  [unwired: 2 in, 2 out]
            n182 = Number To Decimal String(number=w454, width (-)=i16 2) -> (decimal integer string=w449:string)
            n183 = Wait (ms)(milliseconds to wait=u32 500) -> ()  [unwired: 1 out]
            n184 = Concatenate Strings("File path for video", "_" ("string"), w449, "Hz.avi" ("string")) -> (w451:string)
            n185 = String To Path(string=w451) -> (path=w452:path)
            n186 = call "IMAQ AVI2 Create"("Codec"="Motion JPEG (NI Vision)", "Frames Per Second"=w454, "AVI Path"=w452) -> ("AVI Refnum"=w456:T11)  [unwired: 7 in, 1 out]
          }
          frame #2 {
          }
          frame #3 {
            n187 = property on="Trigger Laser" class="Bool (strict)"("Val(Sgnl)"=TRUE ("Value (Signaling)")) -> ()  [unwired: 2 in, 2 out]
          }
          frame #4 {
            n188 = while {
              tunnel: w475 -> [w485]
              shift-right: [w483] -> w473
              shift-left: w476 -> [w486]
              shift-right: [w482] -> w472
              shift-left: w474 -> [w484]
              shift-right: [w487] -> w477
              shift-left: w471 -> [w481]
              stop <- w479 stop-if-true
              n189 = call <vilib>:"IMAQdx Grab2.vi"("error in"=w486, "Image In"=w485, "Session In"=w484) -> ("error out"=w483:errorcluster, "Image Out"=w480:T2, "Session Out"=w482:T5)  [unwired: 5 in, 1 out]
              n190 = call "IMAQ AVI2 Write Frame"("Image"=w480, "AVI Refnum"=w481) -> ("AVI Refnum (duplicate)"=w487:T11)  [unwired: 7 in, 2 out]
              n191 = property on="Video" class="Bool (strict)"() -> ("Value"=w478:bool)  [unwired: 2 in, 2 out]
              n192 = Not(x=w478) -> (.not. x?=w479:bool)
            }
          }
          frame #5 {
            n193 = call "IMAQ AVI2 Close"("AVI Refnum"=w488) -> ()  [unwired: 10 in, 1 out]
          }
          frame #6 {
            n194 = property on="ON/OFF" class="Bool (strict)"("Val(Sgnl)"=FALSE ("Value (Signaling)")) -> ()  [unwired: 2 in, 2 out]
          }
          frame #7 {
            n195 = property on="Action" class="LstBox (strict)"("Val(Sgnl)"=0 ("Value (Signaling)")) -> ()  [unwired: 2 in, 2 out]
          }
          frame #8 {
            n196 = property on="Trigger Laser" class="Bool (strict)"("Val(Sgnl)"=FALSE ("Value (Signaling)")) -> ()  [unwired: 2 in, 2 out]
          }
        }
      }
    }
  }
  "error out" <- w50
  n197 = Initialize Array(0.0 ("element"), 1 ("dimension size")) -> (→"varLaplacian":dbl[])
  n198 = Initialize Array(0.0 ("element"), 1 ("dimension size")) -> (→"meanIntensity":dbl[])
  n199 = call <vilib>:"IMAQdx Close Camera.vi"("Session In"=w2) -> ()  [unwired: 10 in, 1 out]
